vi "main.vi"() -> ()   [LabVIEW 2018]
doc: "This example demonstrates the use of binary morphological reconstruction in the particle analysis. The example allows you to keep the particles completely inside the ROI, completely outside the ROI or on the ROI."
uses:
  <vilib>/vision/NI_Vision_Development_Module.lvlib
panel:
  in  "预处理":bool
  in  "条件1-面积判断":T2(array[cluster]) {"Measurement Parameter" items=["Area"]; "下限" min=0 step=1; "上限" min=0 step=1}
  in  "条件2-灰度阈值":cluster{"下限":i32, "上限":i32}={"下限"=128, "上限"=255} {"下限" min=0 max=255 step=1; "上限" min=0 max=255 step=1}
  in  "查看标注":bool
  in  "导入图像":bool
  in  "删除标注":bool
  in  "退出":bool
  out "标注框总数":dbl
  out "全图灰度级信息":T3 {"标准差" format="%.2f"; "均值" format="%.2f"; "相邻灰度级间隔" format="%.2f"; "起始灰度值" format="%.2f"; "最大值" format="%.2f"; "最小值" format="%.2f"}
  out "全图灰度表":u32[](graph)
  in  "Font, Size & Style 2":T4={"Desired Font (Application)"=enum."Application Font", "[User-specified Font]"={"Font Name"="", "Size"=12, "Strikeout?"=FALSE, "Italic?"=FALSE, "Underline?"=FALSE, "Outline?"=FALSE, "Shadow?"=FALSE, "Bold?"=FALSE, "Rotation Angle"=0.0}, "Horizontal Alignment"=0, "Vertical Alignment"=0} {"Vertical Alignment" items=["Bottom", "Top", "Baseline"]; "Horizontal Alignment" items=["Left", "Center", "Right"]; "[User-specified Font]"."Rotation Angle" format="%.2f"}
  in  "Font, Size & Style":T4={"Desired Font (Application)"=enum."Application Font", "[User-specified Font]"={"Font Name"="", "Size"=12, "Strikeout?"=FALSE, "Italic?"=FALSE, "Underline?"=FALSE, "Outline?"=FALSE, "Shadow?"=FALSE, "Bold?"=FALSE, "Rotation Angle"=0.0}, "Horizontal Alignment"=0, "Vertical Alignment"=0} {"Vertical Alignment" items=["Bottom", "Top", "Baseline"]; "Horizontal Alignment" items=["Left", "Center", "Right"]; "[User-specified Font]"."Rotation Angle" format="%.2f"}
  out "框组":T5(array[cluster])
  in  "Operation":enum16{"overlay rectangle"}(ring)
  out "标注图":T6(plugin-control)
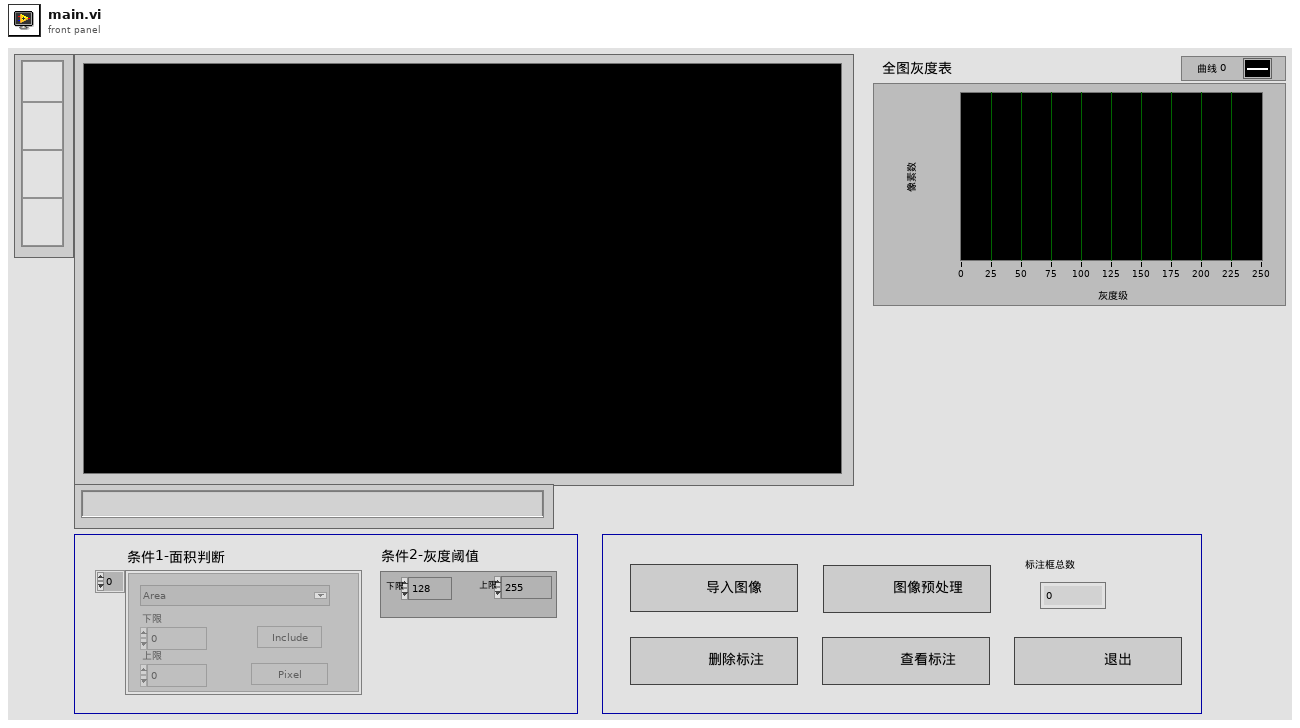
[diagram p1: front panel]
types:
  T1 = typedef "Particle Parameters" = i32
  T2 = cluster{"Measurement Parameter":T1, "下限":i32, "上限":i32, "Range":bool, "Measurement Type":bool}[]
  T3 = cluster{"histogram":u32[], "最小值":sgl, "最大值":sgl, "起始灰度值":sgl, "相邻灰度级间隔":sgl, "均值":sgl, "标准差":sgl, "像素面积":i32}
  T4 = cluster{"Desired Font (Application)":enum16{"User-specified Font", "Application Font", "System Font", "Dialog Font"}, "[User-specified Font]":cluster{"Font Name":string, "Size":i16, "Strikeout?":bool, "Italic?":bool, "Underline?":bool, "Outline?":bool, "Shadow?":bool, "Bold?":bool, "Rotation Angle":dbl}, "Horizontal Alignment":i16, "Vertical Alignment":i16}
  T5 = cluster{"Global Rectangle":i32[], "Contours":cluster{"Contour Type":u32, "ROI Type":u32, "Points":i32[]}[]}[]
  T6 = typedef "IMAQ Image.ctl" = refnum<image>
  T7 = typedef "Image Type" = u32
  T8 = cluster{"Global Rectangle":i32[], "Contours":cluster{"Contour Type":u32, "ROI Type":u32, "Points":i32[]}[]}
  T9 = cluster{"histogram":u32[], "Minimal Value":sgl, "Maximal Value":sgl, "Starting Value":sgl, "Interval Width":sgl, "Mean Value":sgl, "Standard  Variation":sgl, "Area (pixels)":i32}
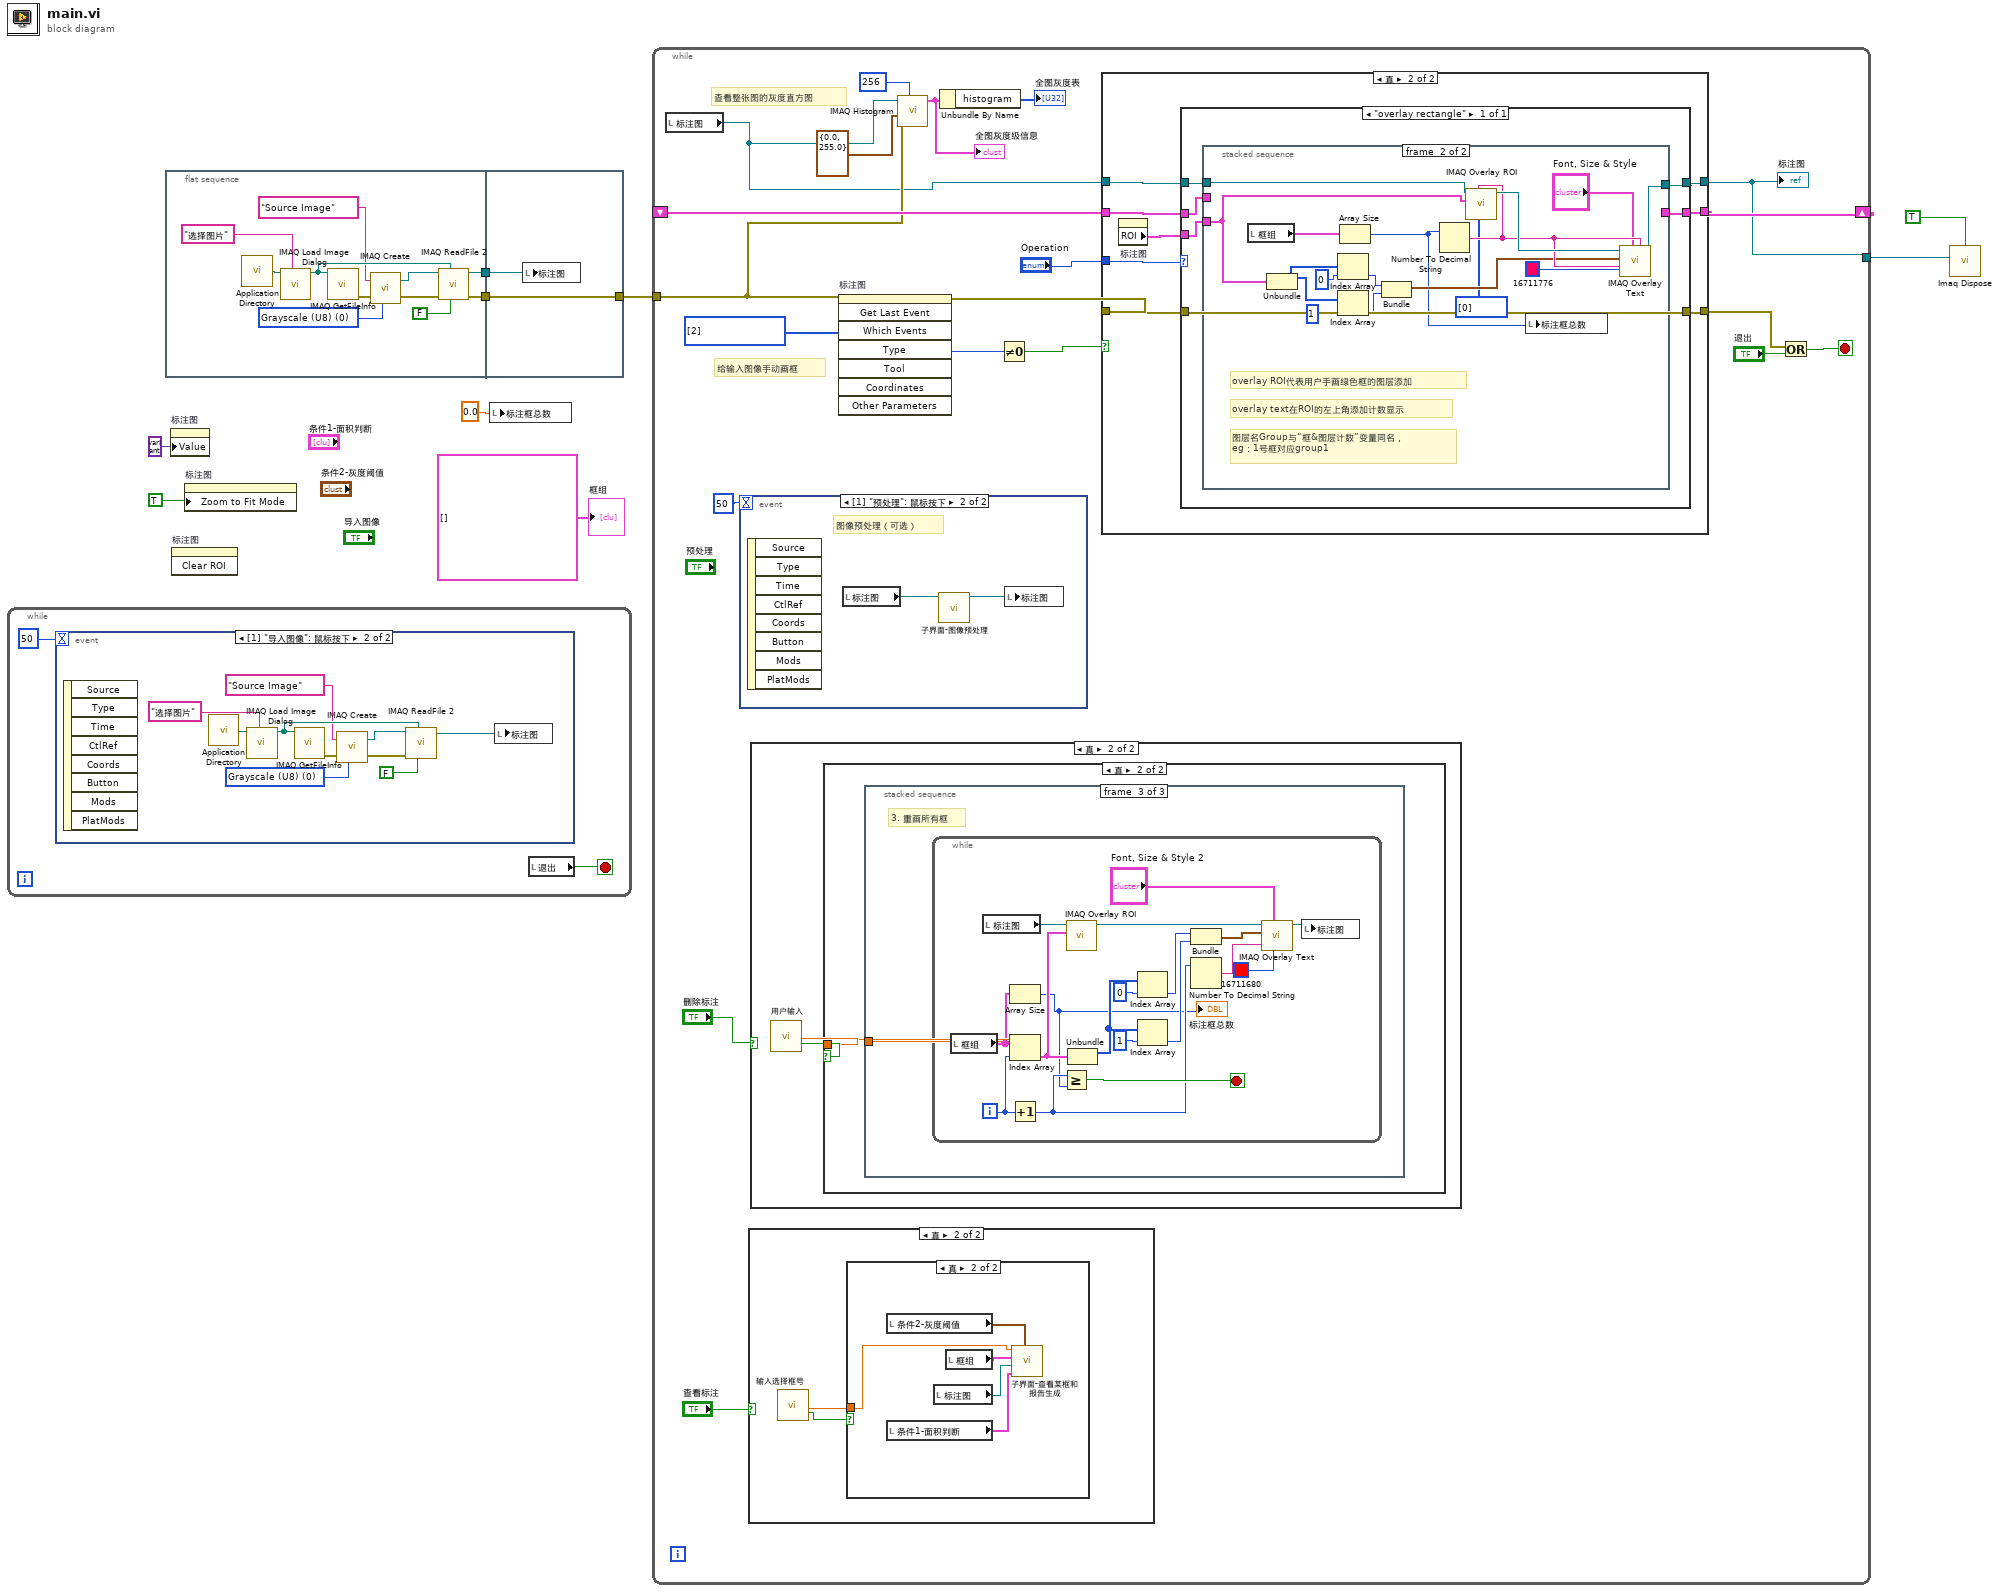
[diagram p0: block diagram]
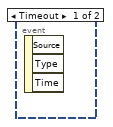
[diagram p2: hidden frame]
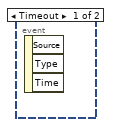
[diagram p3: hidden frame]
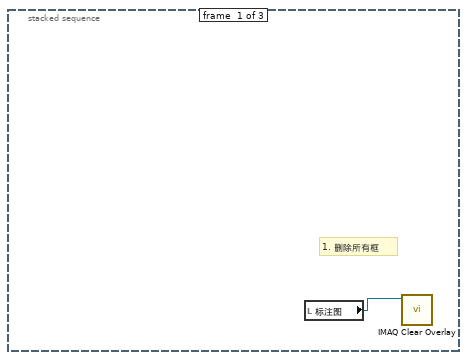
[diagram p8: hidden frame]
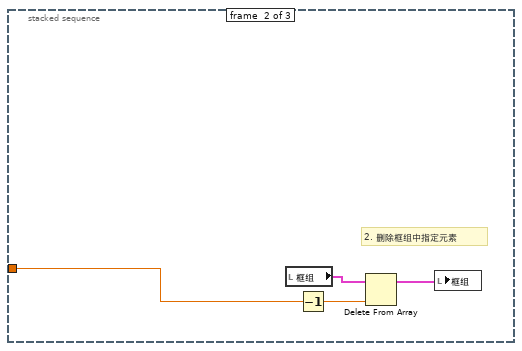
[diagram p9: hidden frame]
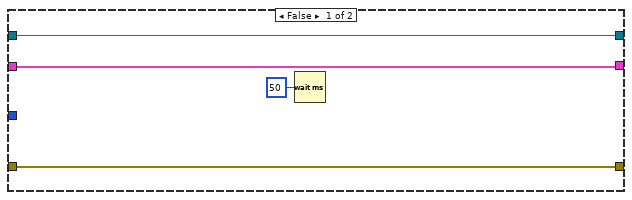
[diagram p10: hidden frame]
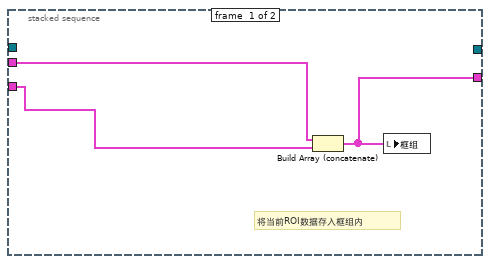
[diagram p11: hidden frame]
diagram:
  n1 = while {
    stop <- w10 stop-if-true
    n2 = event shown="[1] \"导入图像\": 鼠标按下" {
      selector: _ -> [_ _]
      dyn-events: _ -> [_ _]
      timeout: 50 -> [_ _]
      event Timeout {
        n3 = event-data() -> ()  [unwired: 1 in, 3 out]
      }
      event "导入图像": Mouse Down {
        w13 = T7 0 items=["Grayscale (U8)", "Grayscale (I16)", "Grayscale (SGL)", "Complex (CSG)", "RGB (U32)", "HSL (U32)", "RGB (U64)", "Grayscale (U16)"] ("Image Type")
        n4 = event-data() -> ()  [unwired: 1 in, 8 out]
        n5 = call <vilib>:"Application Directory.vi"() -> ("Application Directory"=w21:path)
        n6 = call "IMAQ Load Image Dialog"("Prompt"="选择图片" ("prompt"), "Start Path"=w21) -> ("Path"=w17:path)  [unwired: 7 in, 2 out]
        n7 = call "IMAQ GetFileInfo"("File Path"=w17) -> ("error out"=w18:errorcluster)  [unwired: 4 in, 6 out]
        n8 = call "IMAQ Create"("Image Name"="Source Image", "Image Type"=w13, "error in (no error)"=w18) -> ("New Image"=w19:T6, "error out"=w20:errorcluster)  [unwired: 2 in]
        n9 = call "IMAQ ReadFile 2"("Use File Path Image Type"=FALSE, "File Path"=w17, "error in (no error)"=w20, "Image"=w19) -> ("Image Out"=w12:T6)  [unwired: 3 in, 4 out]
        n10 = local write "标注图"(w12) -> ()
      }
    }
    n11 = local read "退出"() -> (w10:bool)
  }
  n12 = flat-sequence {
    tunnel: [w23] -> w2
    tunnel: [w22] -> w1
    tunnel: [w34] -> w9
    tunnel: w2 -> [w34]
    tunnel: w1 -> [w33]
    frame #0 {
      w24 = T7 0 items=["Grayscale (U8)", "Grayscale (I16)", "Grayscale (SGL)", "Complex (CSG)", "RGB (U32)", "HSL (U32)", "RGB (U64)", "Grayscale (U16)"] ("Image Type")
      n13 = call <vilib>:"Application Directory.vi"() -> ("Application Directory"=w32:path)
      n14 = call "IMAQ Load Image Dialog"("Prompt"="选择图片" ("prompt"), "Start Path"=w32) -> ("Path"=w28:path)  [unwired: 7 in, 2 out]
      n15 = call "IMAQ GetFileInfo"("File Path"=w28) -> ("error out"=w29:errorcluster)  [unwired: 4 in, 6 out]
      n16 = call "IMAQ Create"("Image Name"="Source Image", "Image Type"=w24, "error in (no error)"=w29) -> ("New Image"=w30:T6, "error out"=w31:errorcluster)  [unwired: 2 in]
      n17 = call "IMAQ ReadFile 2"("Use File Path Image Type"=FALSE, "File Path"=w28, "error in (no error)"=w31, "Image"=w30) -> ("error out"=w23:errorcluster, "Image Out"=w22:T6)  [unwired: 3 in, 3 out]
    }
    frame #1 {
      n18 = local write "标注图"(w33) -> ()
    }
  }
  n19 = property on="标注图" class="ImageControl"("Value"=variant ("值")) -> ()  [unwired: 2 in, 2 out]
  n20 = invoke on="标注图" class="ImageControl" method="Clear ROI"() -> ()  [unwired: 3 in, 3 out]
  n21 = property on="标注图" class="ImageControl"("Zoom to Fit Mode"=TRUE) -> ()  [unwired: 2 in, 2 out]
  n22 = local write "标注框总数"(0.0 ("框总数")) -> ()
  n23 = while {
    shift-right: [w47] -> _
    shift-left: _ -> [w46]
    tunnel: w9 -> [w45]
    tunnel: [w37] -> w4
    stop <- w49 stop-if-true
    w52 = i32[] [2] items=["No Event"=0, "Click Event"=1, "Draw Event"=2, "Size Event"=4, "Scroll Event"=5, "Double Click Event"=8] ("Which Events")
    # "给输入图像手动画框"
    # "查看整张图的灰度直方图"
    n24 = local read "标注图"() -> (w38:T6)
    n25 = event shown="[1] \"预处理\": 鼠标按下" {
      selector: _ -> [_ _]
      dyn-events: _ -> [_ _]
      timeout: 50 -> [_ _]
      event Timeout {
        n26 = event-data() -> ()  [unwired: 1 in, 3 out]
      }
      event "预处理": Mouse Down {
        # "图像预处理（可选）"
        n27 = event-data() -> ()  [unwired: 1 in, 8 out]
        n28 = local read "标注图"() -> (w56:T6)
        n29 = call "子界面-图像预处理.vi"("原图"=w56) -> ("处理后"=w55:T6)  [unwired: 10 in]
        n30 = local write "标注图"(w55) -> ()
      }
    }
    n31 = case shown="真" "查看标注" {
      frame False {
      }
      frame True {
        n32 = call "输入选择框号"() -> ("框号"=w58:dbl, "确定"=w57:bool)  [unwired: 17 in, 1 out]
        n33 = case shown="真" w57 {
          tunnel: w58 -> [_ w63]
          frame False {
            # "用户取消操作"
          }
          frame True {
            n34 = local read "条件2-灰度阈值"() -> (w59:cluster{"下限":i32, "上限":i32})
            n35 = local read "条件1-面积判断"() -> (w60:T2)
            n36 = local read "标注图"() -> (w61:T6)
            n37 = local read "框组"() -> (w62:T5)
            n38 = call "子界面-查看某框和报告生成.vi"("条件2-灰度阈值"=w59, "条件1-面积判断"=w60, "标注图"=w61, "框组"=w62, "框号"=w63) -> ()  [unwired: 2 in]
          }
        }
      }
    }
    n39 = case shown="真" "删除标注" {
      frame False {
      }
      frame True {
        n40 = call "用户输入"() -> ("框号"=w64:dbl, "确定"=w65:bool)  [unwired: 17 in, 1 out]
        n41 = case shown="真" w65 {
          tunnel: w64 -> [_ w66]
          frame False {
            # "用户取消操作"
          }
          frame True {
            n42 = stacked-sequence {
              tunnel: w66 -> [_ w70 _]
              frame #0 {
                # "1. 删除所有框"
                n43 = local read "标注图"() -> (w67:T6)
                n44 = call "IMAQ Clear Overlay"("Image"=w67) -> ()  [unwired: 9 in, 2 out]
              }
              frame #1 {
                # "2. 删除框组中指定元素"
                n45 = local read "框组"() -> (w71:T5)
                n46 = Decrement(x=w70) -> (x-1=w69:dbl)
                n47 = Delete From Array(array=w71, index=w69) -> (array with subset deleted=w68:T5)  [unwired: 1 in, 1 out]
                n48 = local write "框组"(w68) -> ()
              }
              frame #2 {
                # "3. 重画所有框"
                n49 = while {
                  i -> [w74]
                  stop <- w89 stop-if-true
                  n50 = local read "框组"() -> (w82:T5)
                  n51 = local read "标注图"() -> (w88:T6)
                  n52 = Array Size(array=w82) -> (size(s)=w72:i32)
                  "标注框总数" <- w72
                  n53 = Index Array(array=w82, index=w74) -> (element=w75:T8)
                  n54 = Increment(x=w74) -> (x+1=w87:i32)
                  n55 = Greater Or Equal?(x=w87, y=w72) -> (x >= y?=w89:bool)
                  n56 = call "IMAQ Overlay ROI"("ROI Descriptor"=w75, "Image"=w88) -> ("Image Out"=w84:T6)  [unwired: 8 in, 1 out]
                  n57 = Unbundle(w75) -> ("Global Rectangle"=w78:i32[])  [unwired: 1 out]
                  n58 = Index Array(array=w78, index=0 ("索引")) -> (element=w79:i32)
                  n59 = Index Array(array=w78, index=1 ("索引")) -> (element=w80:i32)
                  n60 = Bundle(w79, w80) -> (w77:cluster{i32, i32})  [unwired: 1 in]
                  n61 = Number To Decimal String(number=w87) -> (decimal integer string=w85:string)  [unwired: 1 in]
                  n62 = call "IMAQ Overlay Text"("Text Color (black)"=u32 16711680, "Font, Size & Style"="Font, Size & Style 2", "String"=w85, "Origin"=w77, "Image"=w84) -> ("Image Out"=w83:T6)  [unwired: 5 in, 1 out]
                  n63 = local write "标注图"(w83) -> ()
                }
              }
            }
          }
        }
      }
    }
    n64 = invoke on="标注图" class="ImageControl" method="Get Last Event"(error in=w45, "Which Events"=w52) -> (error out=w51:errorcluster, "Type"=w53:i32)  [unwired: 6 in, 6 out]
    n65 = call "IMAQ Histogram"("Number of Classes"=256, "error in (no error)"=w45, "Interval Range"=cluster{"Minimum":sgl, "Maximum":sgl} {"Minimum"=0.0, "Maximum"=255.0}, "Image"=w38) -> ("Histogram Report"=w42:T9)  [unwired: 6 in, 1 out]
    "全图灰度级信息" <- w42
    n66 = Unbundle By Name(w42) -> ("histogram"=→"全图灰度表":u32[])
    n67 = Not Equal To 0?(x=w53) -> (x != 0?=w48:bool)
    n68 = case shown="真" w48 {
      tunnel: w38 -> [w93 w101]
      tunnel: [w93 w100] -> w37
      tunnel: "Operation" -> [_ w98]
      tunnel: w51 -> [w92 w97]
      tunnel: [w92 w96] -> w50
      tunnel: [w90 w95] -> w47
      tunnel: w46 -> [w90 w94]
      frame False {
        n69 = Wait (ms)(milliseconds to wait=u32 50) -> ()  [unwired: 1 out]
      }
      frame True {
        n70 = property on="标注图" class="ImageControl"() -> ("ROI"=w99:T8)  [unwired: 2 in, 2 out]
        n71 = case shown="\"overlay rectangle\"" w98 {
          tunnel: w101 -> [w106]
          tunnel: w99 -> [w104]
          tunnel: [w105] -> w100
          tunnel: w97 -> [w107]
          tunnel: [w107] -> w96
          tunnel: [w103] -> w95
          tunnel: w94 -> [w102]
          frame "overlay rectangle" {
            n72 = stacked-sequence {
              tunnel: w106 -> [_ w117]
              tunnel: [_ w116] -> w105
              tunnel: w104 -> [w110 w113]
              tunnel: [w108 _] -> w103
              tunnel: w102 -> [w109 _]
              frame #0 {
                # "将当前ROI数据存入框组内"
                n73 = Build Array (concatenate)(w109, w110) -> (w108:T5)
                n74 = local write "框组"(w108) -> ()
              }
              frame #1 {
                # "图层名Group与“框&图层计数”变量同名，\neg：1号框对应group1"
                # "overlay text在ROI的左上角添加计数显示"
                # "overlay ROI代表用户手画绿色框的图层添加"
                n75 = local read "框组"() -> (w122:T5)
                n76 = Unbundle(w113) -> ("Global Rectangle"=w125:i32[])  [unwired: 1 out]
                n77 = Index Array(array=w125, index=0 ("索引")) -> (element=w124:i32)
                n78 = Index Array(array=w125, index=1 ("索引")) -> (element=w123:i32)
                n79 = Array Size(array=w122) -> (size(s)=w111:i32)
                n80 = Bundle(w124, w123) -> (w115:cluster{i32, i32})  [unwired: 1 in]
                n81 = Number To Decimal String(number=w111) -> (decimal integer string=w121:string)  [unwired: 1 in]
                n82 = call "IMAQ Overlay ROI"("Colors (Green)"=u32[] [0], "Group"=w121, "ROI Descriptor"=w113, "Image"=w117) -> ("Image Out"=w126:T6)  [unwired: 6 in, 1 out]
                n83 = local write "标注框总数"(w111) -> ()
                n84 = call "IMAQ Overlay Text"("Group"=w121, "Text Color (black)"=u32 16711776, "Font, Size & Style"="Font, Size & Style", "String"=w121, "Origin"=w115, "Image"=w126) -> ("Image Out"=w116:T6)  [unwired: 4 in, 1 out]
              }
            }
          }
        }
      }
    }
    "标注图" <- w37
    n85 = Or(x=w50, y="退出") -> (x .or. y?=w49:bool)
  }
  n86 = call "Imaq Dispose"("All Images? (No)"=TRUE, "Image"=w4) -> ()  [unwired: 1 in, 4 out]
  "框组" <- T5 [] ("框组")
